vi "ReadObjectLayout.vi"(7 "properties to ignore":variant, 8 "error in (no error)":errorcluster, 10 "GObj Refnum":refnum<vi>, 11 "Control Layout in":refnum<class "GraphChart Control Layout.lvclass">) -> (0 "error out":errorcluster, 3 "Control Layout out":refnum<class "GraphChart Control Layout.lvclass">)   [LabVIEW 2010, in "NI_SE_Front Panel Layout.lvlib" / "GraphChart Control Layout.lvclass"]
doc: "Read layout information from the GObj Refnum."
uses:
  GraphChart Control Layout.lvclass
  Control Layout/Control Layout.lvclass
  GraphChart Control Layout.lvclass/GraphChart Control Layout.ctl
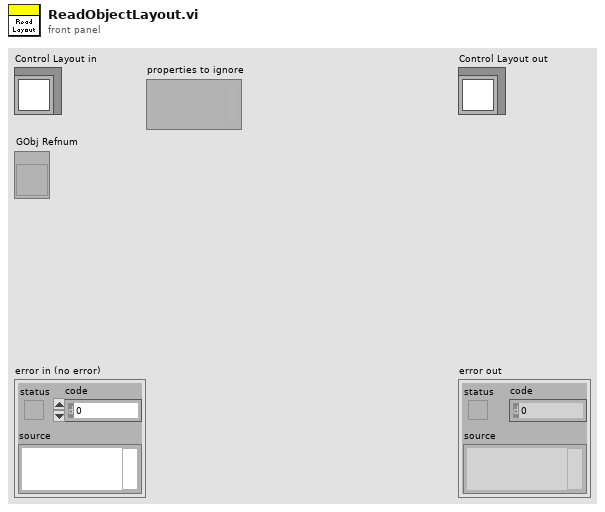
[diagram p1: front panel]
types:
  T1 = typedef "LVRectTypeDef.ctl" = cluster{"left":i16, "top":i16, "right":i16, "bottom":i16}
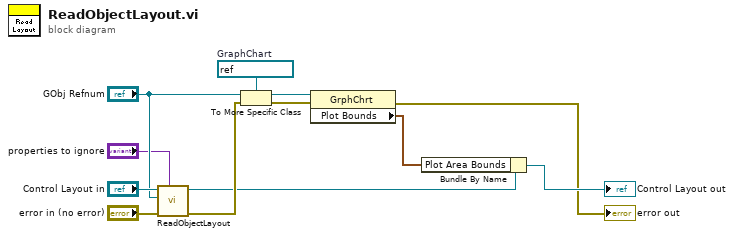
[diagram p0: block diagram]
diagram:
  w4 = refnum<vi> refnum  # GraphChart
  n1 = call-parent "ReadObjectLayout.vi"("properties to ignore"="properties to ignore", "error in (no error)"="error in (no error)", "GObj Refnum"="GObj Refnum", "Control Layout in"="Control Layout in") -> ("error out"=w10:errorcluster, "Control Layout out"=w9:refnum<class "GraphChart Control Layout.lvclass">)  [unwired: 6 in]
  n2 = To More Specific Class(target class=w4, reference="GObj Refnum", error in=w10) -> (specific class reference=w2:refnum<vi>, error out=w3:errorcluster)
  n3 = property class="GrphChrt"(reference=w2, error in=w3) -> (error out=→"error out":errorcluster, "Plot Bounds"=w1:T1)  [unwired: 1 out]
  n4 = Bundle By Name(cluster=w9, "Plot Area Bounds"=w1) -> (→"Control Layout out":refnum<class "GraphChart Control Layout.lvclass">)
